vi "sendVSSRefPlacement.vi"(5 "VSSRef Replacement infos":T6={"Local IP:"="192.168.0.102", "Port"=10003, "Server IP:"="224.5.23.2"}, 8 "x .and. y?":bool, 9 "color":enum16{"Azul", "Amarelo"}(ring), 10 "RobotPlacement":T5(array[cluster])) -> ()   [LabVIEW 2020]
uses:
  Controls/vision_control.ctl
  Paths/Convert AI Robot to Robot Command Folder/grSim/grSim Robot Command.ctl
  Paths/grSim Packet Command UDP Test Folder/grSim/grSim RobotReplacement.ctl
  Paths/grSim Packet Command UDP Test Folder/grSim/grSim_BallReplacement.ctl
  Paths/MessageAI_State Folder/Varint Encoder uint32.vi
panel:
  in  "FIRASim?":bool=TRUE
  in  "grSim replacement":T3={"grSim_RobotReplacement"=[{"x"=0.0, "y"=-450.0, "dir"=0.0, "yellowteam"=FALSE, "id"=0}, {"x"=0.0, "y"=-270.0, "dir"=0.0, "yellowteam"=FALSE, "id"=1}, {"x"=0.0, "y"=-90.0, "dir"=0.0, "yellowteam"=FALSE, "id"=2}, {"x"=0.0, "y"=90.0, "dir"=0.0, "yellowteam"=FALSE, "id"=3}, {"x"=0.0, "y"=270.0, "dir"=0.0, "yellowteam"=FALSE, "id"=4}, {"x"=0.0, "y"=450.0, "dir"=0.0, "yellowteam"=FALSE, "id"=5}], "grSim_BallReplacement"={"x"=0.0, "y"=0.0, "vx"=0.0, "vy"=0.0}}
  in  "replace ball":bool
  out "error out":errorcluster
  out "Array":u8[](array[numeric]) format="%02x"
  in  "isteamyellow":bool=TRUE
  in  "Robots":T4[](array[typedef])
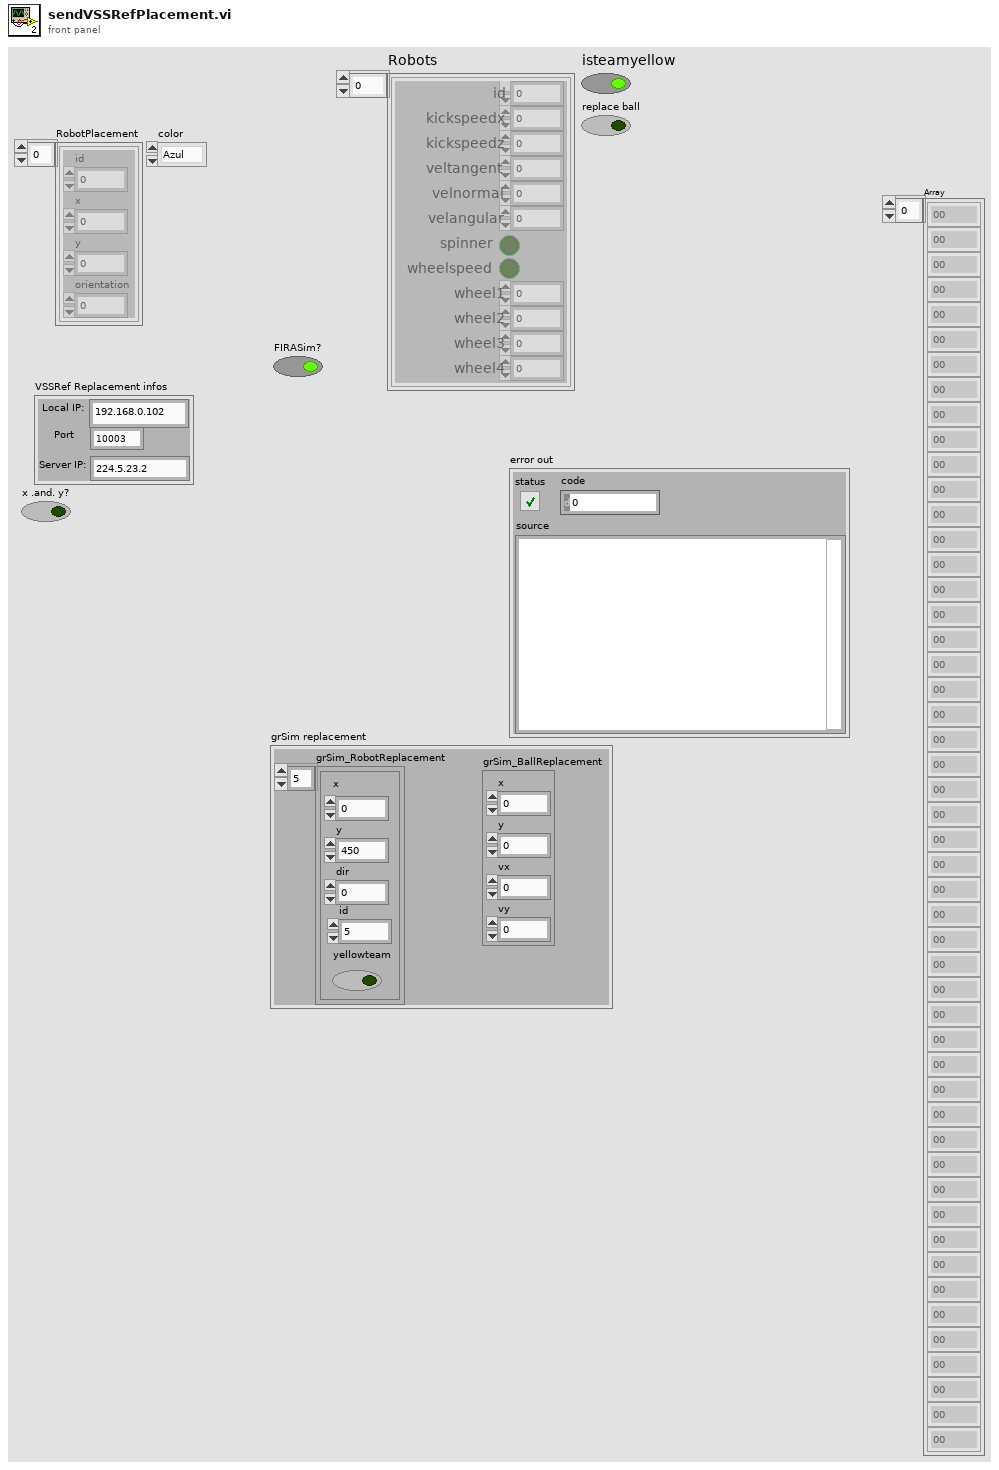
[diagram p1: front panel]
types:
  T1 = typedef "grSim RobotReplacement.ctl" = cluster{"x":dbl, "y":dbl, "dir":dbl, "yellowteam":bool, "id":u32}
  T2 = typedef "grSim_BallReplacement.ctl" = cluster{"x":dbl, "y":dbl, "vx":dbl, "vy":dbl}
  T3 = cluster{"grSim_RobotReplacement":T1[], "grSim_BallReplacement":T2}
  T4 = typedef "grSim Robot Command.ctl" = cluster{"id":u32, "kickspeedx":sgl, "kickspeedz":sgl, "veltangent":sgl, "velnormal":sgl, "velangular":sgl, "spinner":bool, "wheelspeed":bool, "wheel1":sgl, "wheel2":sgl, "wheel3":sgl, "wheel4":sgl}
  T5 = cluster{"id":i32, "x":dbl, "y":dbl, "orientation":dbl}[]
  T6 = typedef "vision_control.ctl" = cluster{"Local IP:":string, "Port":i32, "Server IP:":string}
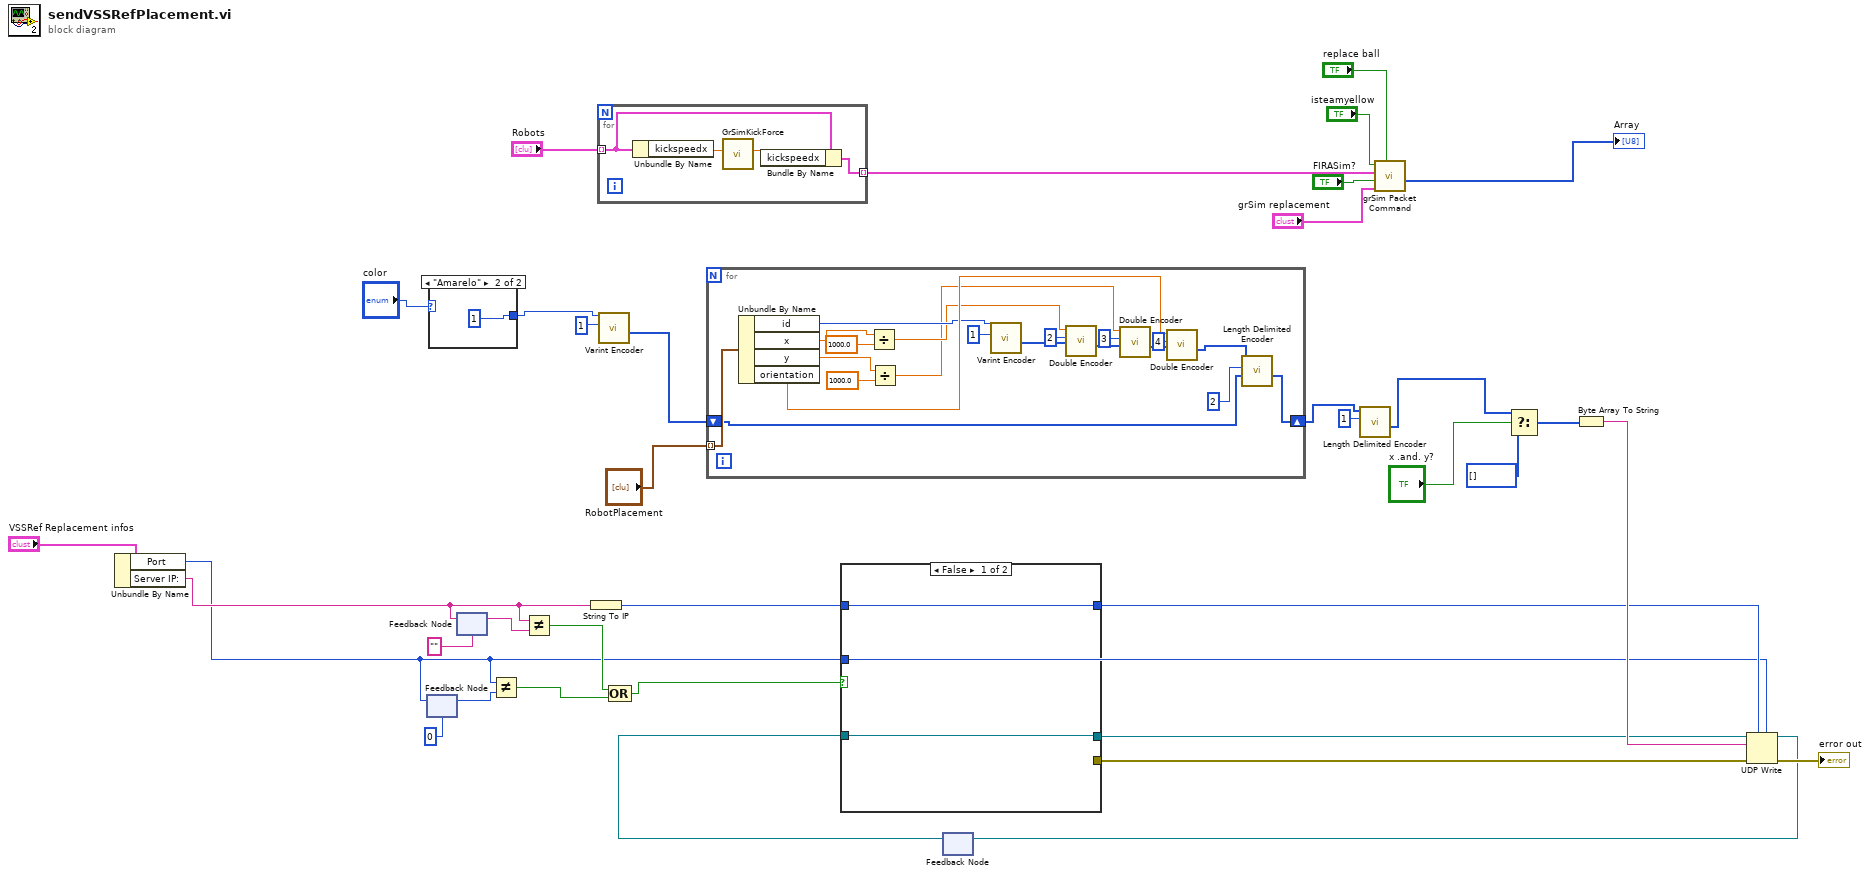
[diagram p0: block diagram]
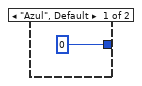
[diagram p2: hidden frame]
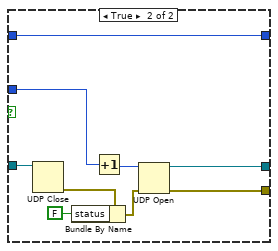
[diagram p3: hidden frame]
diagram:
  n1 = Unbundle By Name("VSSRef Replacement infos") -> ("Port"=w12:i32, "Server IP:"=w13:string)
  n2 = feedback #1(u16 0 ("Port:")) -> (w33:i32)
  n3 = feedback-in #1(w12) -> ()
  n4 = case shown="\"Amarelo\"" "color" {
    tunnel: [0 1] -> w9
    frame "Azul", Default {
    }
    frame "Amarelo" {
    }
  }
  n5 = feedback #2("" ("SSL Vision Address:")) -> (w32:string)
  n6 = feedback-in #2(w13) -> ()
  n7 = Not Equal?(x=w12, y=w33) -> (x != y?=w30:bool)
  n8 = Not Equal?(x=w13, y=w32) -> (x != y?=w31:bool)
  n9 = String To IP(1:w13) -> (0:w22:u32)
  n10 = for {
    tunnel: "Robots" -> [w42] mode=indexing
    tunnel: [w41] -> w19 mode=indexing
    n11 = Unbundle By Name(w42) -> ("kickspeedx"=w40:sgl)
    n12 = call "GrSimKickForce.vi"("real kick"=w40) -> ("grsim kick"=w39:dbl)  [unwired: 10 in]
    n13 = Bundle By Name(cluster=w42, "kickspeedx"=w39) -> (w41:T4)
  }
  n14 = call-poly "Varint Encoder.vi"("Key"=u32 1, "Value"=w9) -> ("Array"=w7:u8[])  [unwired: 9 in]
  n15 = Compound Arithmetic op=OR(w31, w30) -> (w29:bool)
  n16 = for {
    tunnel: "RobotPlacement" -> [w62] mode=indexing
    shift-right: [w51] -> w5
    shift-left: w7 -> [w50]
    n17 = Unbundle By Name(w62) -> ("id"=w49:i32, "x"=w47:dbl, "y"=w44:dbl, "orientation"=w55:dbl)
    n18 = Divide(x=w47, y=1000.0) -> (x/y=w46:dbl)
    n19 = Divide(x=w44, y=1000.0) -> (x/y=w43:dbl)
    n20 = call-poly "Varint Encoder.vi"("Key"=u32 1, "Value"=w49) -> ("Array"=w60:u8[])  [unwired: 9 in]
    n21 = call "Double Encoder.vi"("Array In"=w60, "Key"=u32 2, "Value"=w46) -> ("Array"=w58:u8[])  [unwired: 8 in]
    n22 = call "Double Encoder.vi"("Array In"=w58, "Key"=u32 3, "Value"=w43) -> ("Array"=w56:u8[])  [unwired: 8 in]
    n23 = call "Double Encoder.vi"("Array In"=w56, "Key"=u32 4, "Value"=w55) -> ("Array"=w52:u8[])  [unwired: 8 in]
    n24 = call "Length Delimited Encoder.vi"("Array In"=w50, "Key"=u32 2, "Array In 2"=w52) -> ("Array"=w51:u8[])  [unwired: 8 in]
  }
  n25 = feedback #3() -> (w27:refnum<k16>)  [unwired: 1 in]
  n26 = case shown="False" w29 {
    tunnel: [_ w73] -> w34
    tunnel: [w64 w71] -> w26
    tunnel: w12 -> [_ w70]
    tunnel: w22 -> [w63 w68]
    tunnel: w27 -> [w64 w69]
    tunnel: [w63 w68] -> w21
    frame False {
    }
    frame True {
      n27 = UDP Close(connection ID=w69) -> (error out=w67:errorcluster)  [unwired: 1 in, 1 out]
      n28 = Bundle By Name(cluster=w67, "status"=FALSE) -> (w66:errorcluster)
      n29 = Increment(x=w70) -> (x+1=w72:i32)
      n30 = UDP Open(8:w66, 11:w72) -> (port=w71:refnum<k16>, 0:w73:errorcluster)  [unwired: 3 in, 1 out]
    }
  }
  n31 = call "Length Delimited Encoder.vi"("Key"=u32 1, "Array In 2"=w5) -> ("Array"=w3:u8[])  [unwired: 9 in]
  n32 = call "grSim Packet Command.vi"("replace ball"="replace ball", "grSim replacement"="grSim replacement", "FIRASim?"="FIRASim?", "Robots"=w19, "isteamyellow"="isteamyellow") -> ("Array"=→"Array":u8[])  [unwired: 6 in]
  n33 = Select(t=w3, s="x .and. y?", f=u8[] []) -> (s? t:f=w1:u8[])
  n34 = Byte Array To String(unsigned byte array=w1) -> (string=w35:string)
  n35 = UDP Write(address=w21, port or service name=w12, connection ID=w26, data in=w35, 8:w34) -> (error out=→"error out":errorcluster, 3:w25:refnum<k16>)  [unwired: 1 in]
  n36 = feedback-in #3(w25) -> ()
